vi "Write Self Attributes.vi"(10 "Self Attributes":refnum<class "Attributes.lvclass">, 11 "Actor in":refnum<class "Actor.lvclass">) -> (3 "Actor out":refnum<class "Actor.lvclass">)   [LabVIEW 2020, in "jettl.lvlib" / "Actor.lvclass"]
uses:
  Actor.lvclass
  Attributes/Attributes.lvclass
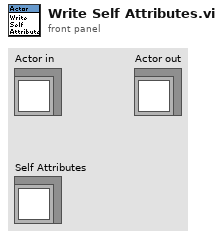
[diagram p1: front panel]
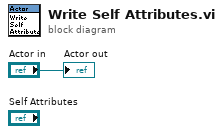
[diagram p0: block diagram]
diagram:
  "Actor out" <- "Actor in"
